vi "proiect.vi"() -> ()   [LabVIEW 2024]
uses:
  <vilib>/DAQmx/read.llb/DAQmx Read (Counter DBL 1Chan 1Samp).vi
  <vilib>/DAQmx/create/channels.llb/DAQmx Create Channel (CI-Count Edges).vi
  <vilib>/DAQmx/miscellaneous.llb/DAQmx Fill In Error Info.vi
  <resource>/objmgr/daqmx.rc
panel:
  out "Gama de masura":string
  in  "Scala":i32(slide) scale=1.0..4.0
  out "Frecventa":dbl
  out "Capacitate":string
  out "String":string
  in  "Delay in milisecunde":u32
  in  "CI.CountEdges.Term":tag
  in  "counter":tag
  in  "stop":bool
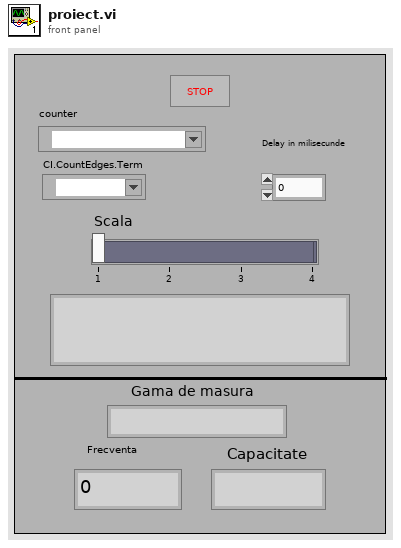
[diagram p1: front panel]
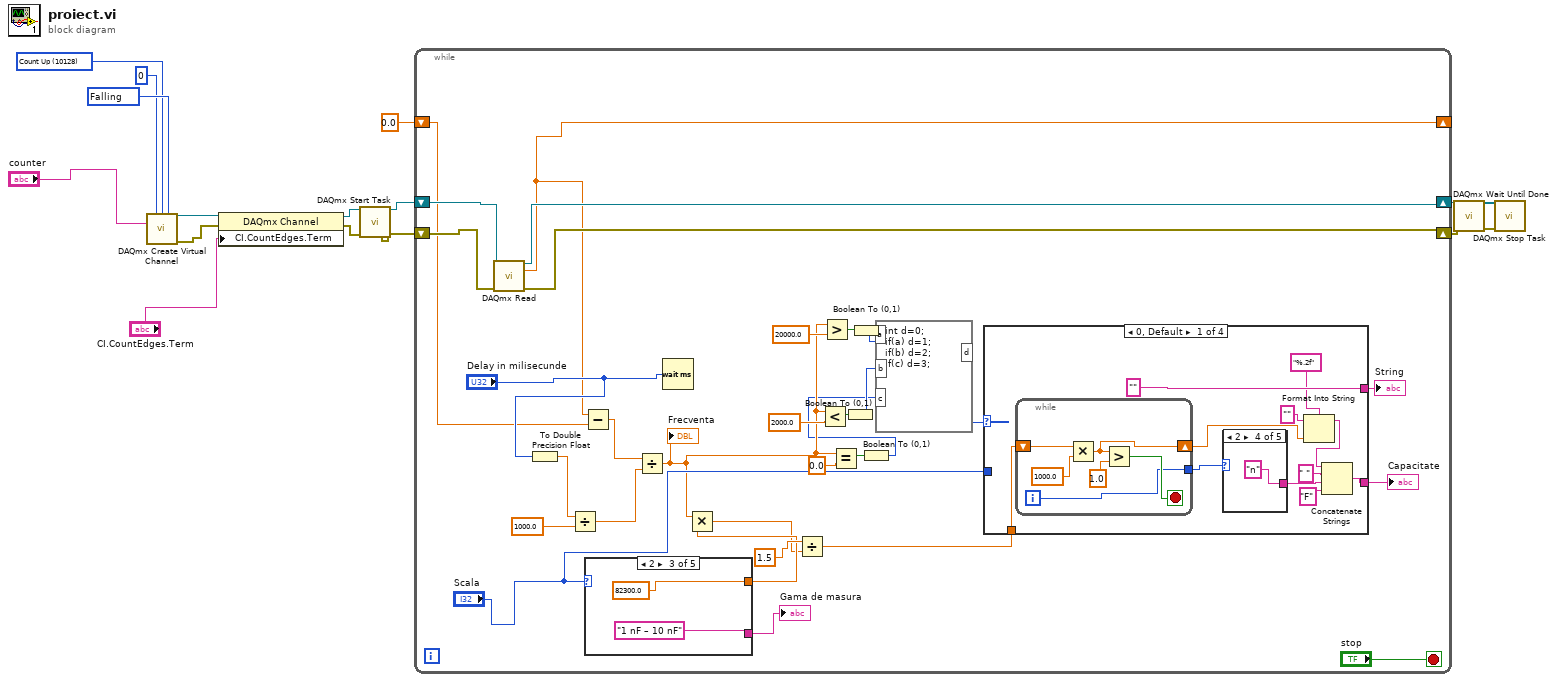
[diagram p0: block diagram]
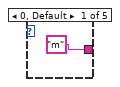
[diagram p2: hidden frame]
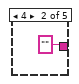
[diagram p3: hidden frame]
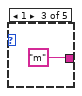
[diagram p4: hidden frame]
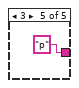
[diagram p5: hidden frame]
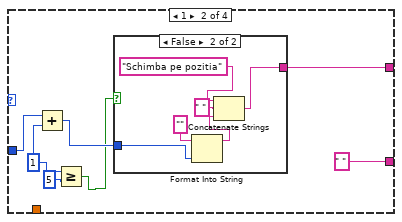
[diagram p6: hidden frame]
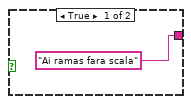
[diagram p7: hidden frame]
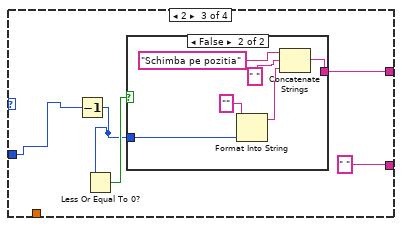
[diagram p8: hidden frame]
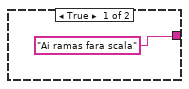
[diagram p9: hidden frame]
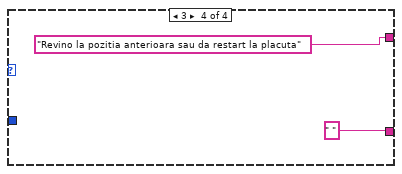
[diagram p10: hidden frame]
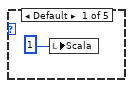
[diagram p11: hidden frame]
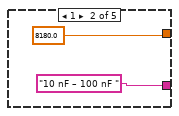
[diagram p12: hidden frame]
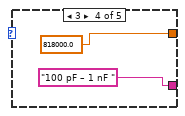
[diagram p13: hidden frame]
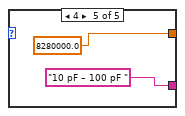
[diagram p14: hidden frame]
diagram:
  w16 = 10171 items=["Rising"=10280, "Falling"=10171] ("edge")
  w15 = 10128 items=["Count Up"=10128, "Count Down"=10124, "Externally Controlled"=10326] ("count direction")
  n1 = call-poly <vilib>:"DAQmx Create Virtual Channel.vi"("initial count"=u32 0, "count direction"=w15, "edge"=w16, "counter"="counter") -> ("task out"=w6:refnum<k21>, "error out"=w5:errorcluster)  [unwired: 10 in]
  n2 = property on="Property Node" class="DAQmx Channel"(reference=w6, error in=w5, "CI.CountEdges.Term"="CI.CountEdges.Term") -> (reference out=w8:refnum<k21>, error out=w7:errorcluster)
  n3 = call <vilib>:"DAQmx Start Task.vi"("task/channels in"=w8, "error in"=w7) -> ("task out"=w9:refnum<k21>, "error out"=w1:errorcluster)  [unwired: 12 in]
  n4 = while {
    shift-right: [w46] -> w13
    shift-left: w9 -> [w47]
    shift-right: [w45] -> w12
    shift-left: w1 -> [w44]
    shift-right: [w22] -> _
    shift-left: 0.0 ("data") -> [w23]
    stop <- "stop" stop-if-true
    n5 = call-poly <vilib>:"DAQmx Read.vi"("task/channels in"=w47, "error in"=w44) -> ("task out"=w46:refnum<k21>, "data"=w22:dbl, "error out"=w45:errorcluster)  [unwired: 11 in]
    n6 = To Double Precision Float(number="Delay in milisecunde") -> (double precision float=w38:dbl)
    n7 = Divide(x=w38, y=1000.0) -> (x/y=w42:dbl)
    n8 = Subtract(x=w22, y=w23) -> (x-y=w24:dbl)
    n9 = case shown="2" "Scala" {
      tunnel: [_ 8180.0 82300.0 818000.0 8280000.0] -> w40
      tunnel: [_ "10 nF – 100 nF " "1 nF – 10 nF" "100 pF – 1 nF " "10 pF – 100 pF "] -> w17
      frame Default {
        n10 = local write "Scala"(1) -> ()
      }
      frame 1 {
      }
      frame 2 {
      }
      frame 3 {
      }
      frame 4 {
      }
    }
    "Gama de masura" <- w17
    n11 = Divide(x=w24, y=w42) -> (x/y=w21:dbl)
    "Frecventa" <- w21
    n12 = Wait (ms)(milliseconds to wait="Delay in milisecunde") -> ()  [unwired: 1 out]
    n13 = Multiply(x=w21, y=w40) -> (x*y=w39:dbl)
    n14 = Divide(x=1.5 ("y"), y=w39) -> (x/y=w26:dbl)
    n15 = Less?(x=w21, y=2000.0) -> (x < y?=w31:bool)
    n16 = Greater?(x=w21, y=20000.0) -> (0:w33:bool)
    n17 = Equal?(x=w21, y=0.0) -> (x = y?=w19:bool)
    n18 = Boolean To (0,1)(Boolean=w31) -> (0, 1=w30:i16)
    n19 = Boolean To (0,1)(Boolean=w33) -> (0, 1=w32:i16)
    n20 = Boolean To (0,1)(Boolean=w19) -> (0, 1=w18:i16)
    n21 = formula code="int d=0;\nif(a) d=1;\nif(b) d=2;\nif(c) d=3;"("a"=w32, "b"=w30, "c"=w18) -> ("d"=w29:i32)
    n22 = case shown="0, Default" w29 {
      tunnel: ["" w76 w88 "Revino la pozitia anterioara sau da restart la placuta"] -> w28
      tunnel: "Scala" -> [_ w73 w84 _]
      tunnel: w26 -> [w57 _ _ _]
      tunnel: [w49 " " " " " "] -> w27
      frame 0, Default {
        n23 = while {
          shift-right: [w64] -> w55
          shift-left: w57 -> [w69]
          tunnel: [w65] -> w56
          i -> [w65]
          stop <- w66 stop-if-true
          n24 = Multiply(x=w69, y=1000.0) -> (x*y=w64:dbl)
          n25 = Greater?(x=w64, y=1.0) -> (0:w66:bool)
        }
        n26 = case shown="2" w56 {
          tunnel: ["m" "" "m" "n" "p"] -> w51
          frame 0, Default {
          }
          frame 4 {
          }
          frame 1 {
          }
          frame 2 {
          }
          frame 3 {
          }
        }
        n27 = Format Into String(format string="%.2f", initial string="", w55) -> (resulting string=w53:string)  [unwired: 1 in, 1 out]
        n28 = Concatenate Strings(w53, " " ("string"), w51, "F" ("string")) -> (w49:string)
      }
      frame 1 {
        w72 = 1 ("y")
        n29 = Add(x=w73, y=w72) -> (x+y=w74:i32)
        n30 = Greater Or Equal?(x=w72, y=5) -> (x >= y?=w70:bool)
        n31 = case shown="False" w70 {
          tunnel: ["Ai ramas fara scala" w83] -> w76
          tunnel: w74 -> [_ w78]
          frame True {
          }
          frame False {
            n32 = Format Into String(initial string="", w78) -> (resulting string=w80:string)  [unwired: 2 in, 1 out]
            n33 = Concatenate Strings("Schimba pe pozitia" ("String"), " " ("string"), w80) -> (w83:string)
          }
        }
      }
      frame 2 {
        n34 = Decrement(x=w84) -> (x-1=w85:i32)
        n35 = Less Or Equal To 0?(x=w85) -> (x <= 0?=w86:bool)
        n36 = case shown="False" w86 {
          tunnel: w85 -> [_ w95]
          tunnel: ["Ai ramas fara scala" w92] -> w88
          frame True {
          }
          frame False {
            n37 = Format Into String(initial string="", w95) -> (resulting string=w91:string)  [unwired: 2 in, 1 out]
            n38 = Concatenate Strings("Schimba pe pozitia" ("String"), " " ("string"), w91) -> (w92:string)
          }
        }
      }
      frame 3 {
      }
    }
    "String" <- w28
    "Capacitate" <- w27
  }
  n39 = call <vilib>:"DAQmx Wait Until Done.vi"("task/channels in"=w13, "error in"=w12) -> ("task out"=w11:refnum<k21>, "error out"=w10:errorcluster)  [unwired: 12 in]
  n40 = call <vilib>:"DAQmx Stop Task.vi"("task/channels in"=w11, "error in"=w10) -> ()  [unwired: 12 in, 2 out]
